vi "Parse.vi"(8 "Error In":errorcluster, 11 "object in":refnum<class "2021_12.lvclass">) -> (0 "Error Out":errorcluster, 3 "object out":refnum<class "2021_12.lvclass">)   [LabVIEW 2020, in "2021_12.lvclass"]
uses:
  2021_12.lvclass
  12_Cave_class/12_Cave.lvclass
  <vilib>/Utility/miscctls.llb/LVMapReplaceAction.ctl
  2021_12.lvclass/2021_12.ctl
panel:
  out "Array":string[][](array[string])
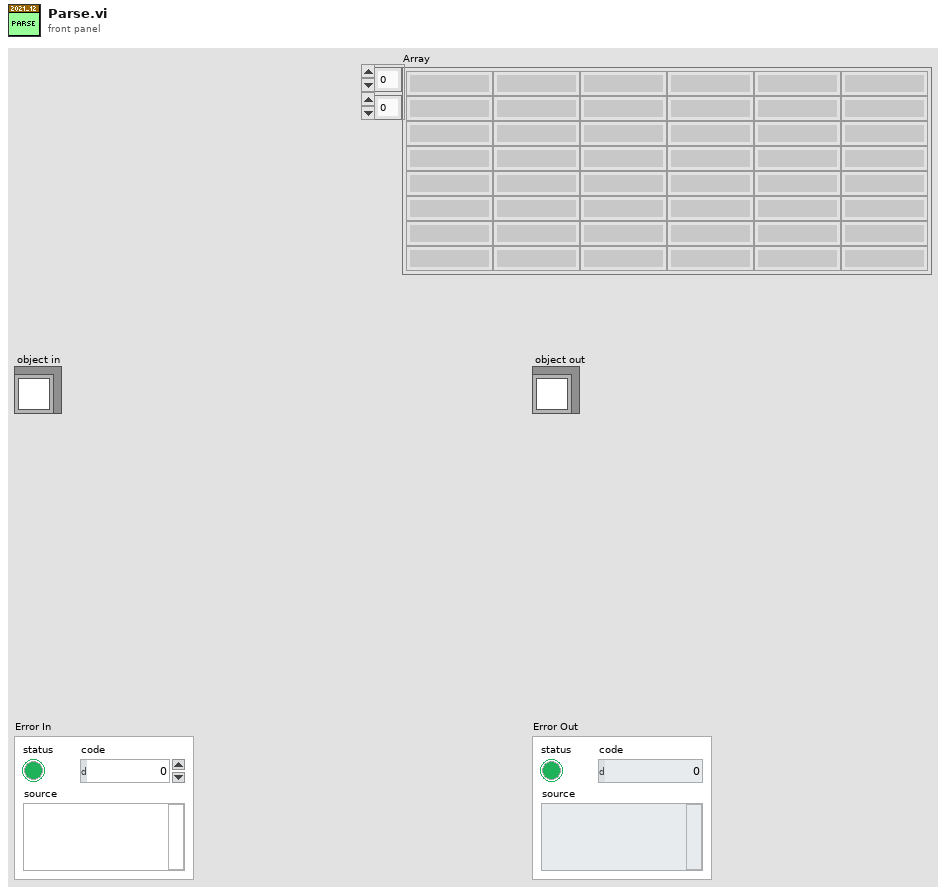
[diagram p1: front panel]
types:
  T1 = typedef "LVMapReplaceAction.ctl" = enum32{"Modify Entry only if found", "Add or Modify Entry", "Delete Entry"}
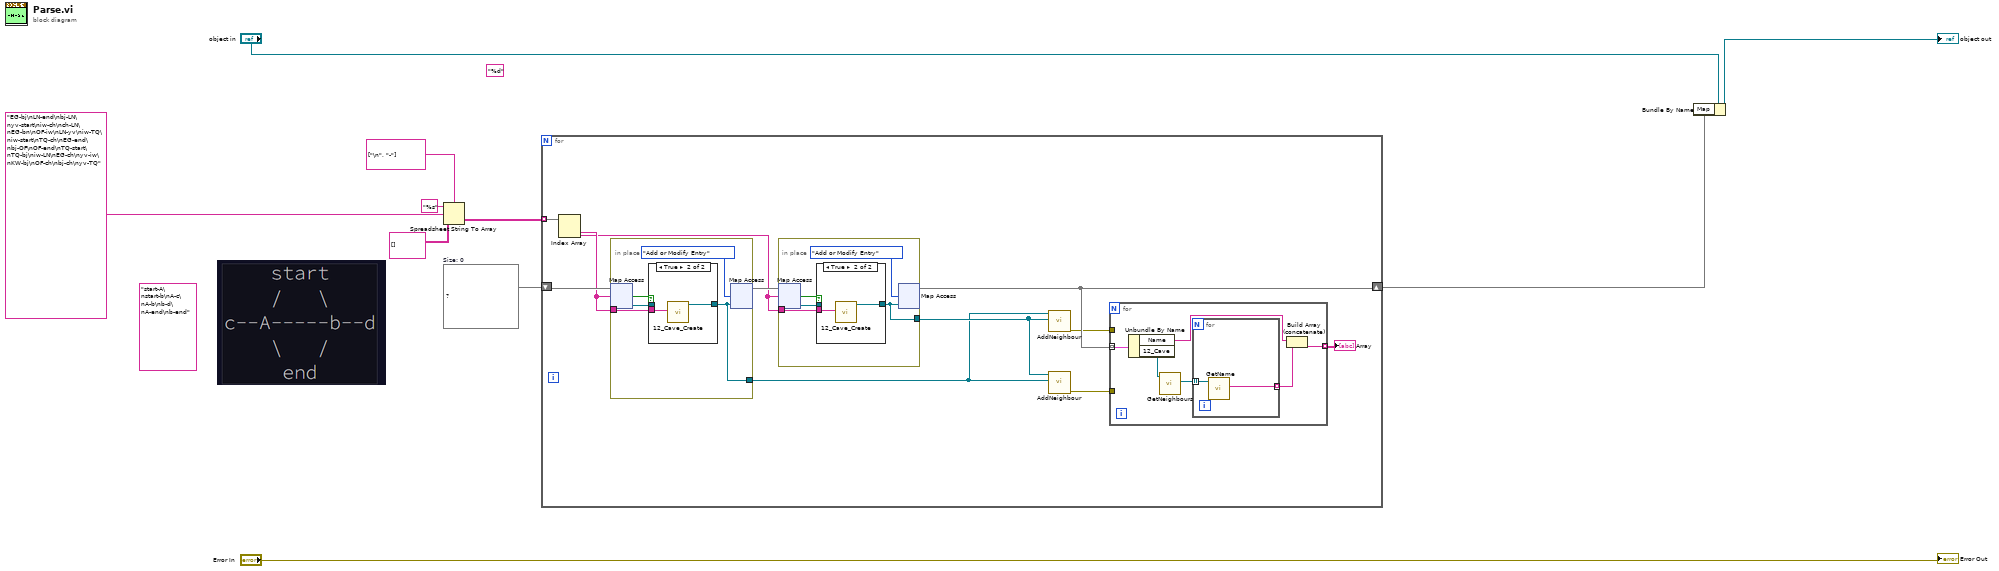
[diagram p0: block diagram]
diagram:
  (unwired) "start-A\nstart-b\nA-c\nA-b\nb-d\nA-end\nb-end" ("PuzzleInput")
  w4 = map{string, refnum<class "12_Cave.lvclass">} {}  # Size: 0
  (unwired) "%d" ("format string")
  n1 = Spreadsheet String To Array(delimiter (Tab)=string[] ["\n", "-"], format string="%s", spreadsheet string="EG-bj\nLN-end\nbj-LN\nyv-start\niw-ch\nch-LN\nEG-bn\nOF-iw\nLN-yv\niw-TQ\niw-start\nTQ-ch\nEG-end\nbj-OF\nOF-end\nTQ-start\nTQ-bj\niw-LN\nEG-ch\nyv-iw\nKW-bj\nOF-ch\nbj-ch\nyv-TQ" ("PuzzleInput"), array type (2D Dbl)=string[][] []) -> (array=w3:string[][])
  n2 = for {
    shift-right: [w13] -> w2
    shift-left: w4 -> [w20]
    tunnel: w3 -> [w21] mode=indexing
    n3 = Index Array(array=w21) -> (element #1=w17:string, element #2=w16:string)  [unwired: 2 in]
    n4 = in-place {
      in-place-border: [w39] -> w15
      in-place-border: w17 -> [w38]
      n5 = in-place-map #1(w20, w17) -> (w41:refnum<class "12_Cave.lvclass">, w42:bool)  [unwired: 1 in]
      n6 = case shown="True" w42 {
        tunnel: w41 -> [w43 _]
        tunnel: [w43 w45] -> w39
        tunnel: w38 -> [_ w44]
        frame False {
        }
        frame True {
          n7 = call "12_Cave_Create.vi"("Name"=w44) -> ("reference out"=w45:refnum<class "12_Cave.lvclass">)  [unwired: 9 in, 1 out]
        }
      }
      n8 = in-place-map #1(w39, LVMapReplaceAction."Add or Modify Entry" ("action")) -> (w19:map{string, refnum<class "12_Cave.lvclass">})  [unwired: 2 out]
    }
    n9 = in-place {
      in-place-border: [w31] -> w18
      in-place-border: w16 -> [w30]
      n10 = in-place-map #2(w19, w16) -> (w33:refnum<class "12_Cave.lvclass">, w34:bool)  [unwired: 1 in]
      n11 = case shown="True" w34 {
        tunnel: w33 -> [w35 _]
        tunnel: [w35 w37] -> w31
        tunnel: w30 -> [_ w36]
        frame False {
        }
        frame True {
          n12 = call "12_Cave_Create.vi"("Name"=w36) -> ("reference out"=w37:refnum<class "12_Cave.lvclass">)  [unwired: 9 in, 1 out]
        }
      }
      n13 = in-place-map #2(w31, LVMapReplaceAction."Add or Modify Entry" ("action")) -> (w13:map{string, refnum<class "12_Cave.lvclass">})  [unwired: 2 out]
    }
    n14 = call-dynamic "AddNeighbour.vi"("Neighbour"=w18, "reference in"=w15) -> ("Error Out"=w12:errorcluster)  [unwired: 8 in, 1 out]
    n15 = call-dynamic "AddNeighbour.vi"("Neighbour"=w15, "reference in"=w18) -> ("Error Out"=w11:errorcluster)  [unwired: 8 in, 1 out]
    n16 = for {
      tunnel: w13 -> [w27] mode=indexing
      tunnel: [w22] -> w14 mode=indexing
      tunnel: w12 -> [_]
      tunnel: w11 -> [_]
      n17 = Unbundle By Name(w27) -> ("Name"=w24:string, "12_Cave"=w26:refnum<class "12_Cave.lvclass">)
      n18 = call-dynamic "GetNeighbours.vi"("reference in"=w26) -> ("Neighbours"=w25:refnum<class "12_Cave.lvclass">[])  [unwired: 8 in, 2 out]
      n19 = for {
        tunnel: w25 -> [w29] mode=indexing
        tunnel: [w28] -> w23 mode=indexing
        n20 = call-dynamic "GetName.vi"("reference in"=w29) -> ("Name"=w28:string)  [unwired: 8 in, 2 out]
      }
      n21 = Build Array (concatenate)(w24, w23) -> (w22:string[])
    }
    "Array" <- w14
  }
  n22 = Bundle By Name(cluster="object in", "Map"=w2) -> (→"object out":refnum<class "2021_12.lvclass">)
  "Error Out" <- "Error In"
